vi "KH TURCK ETHERNETIP RFID UserCommand Read.vi"(8 "index":i32, 11 "Channel":u16) -> (3 "UserCommand":T1=enum."idle")   [LabVIEW 2021]
uses:
  KH TURCK ETHERNETIP TDef Enum RFID User Command.ctl
  KH TURCK ETHERNETIP RFID Global.vi
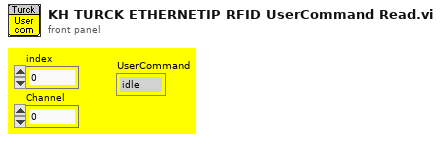
[diagram p1: front panel]
types:
  T1 = typedef "KH TURCK ETHERNETIP TDef Enum RFID User Command.ctl" = enum16{"read", "write", "idle", "inventory"}
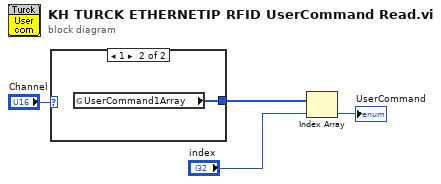
[diagram p0: block diagram]
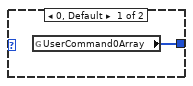
[diagram p2: hidden frame]
diagram:
  n1 = case shown="1" "Channel" {
    tunnel: [w5 w6] -> w4
    frame 0, Default {
      n2 = global read "KH TURCK ETHERNETIP RFID Global.vi" "UserCommand0Array"() -> (w5:T1[])
    }
    frame 1 {
      n3 = global read "KH TURCK ETHERNETIP RFID Global.vi" "UserCommand1Array"() -> (w6:T1[])
    }
  }
  n4 = Index Array(array=w4, index="index") -> (element=→"UserCommand":T1)
